vi "Power Output System Warning.vi"(6 "Driver Ref (null)":T10, 7 "Coerced PV Test Parameters":T1={"Stimulus"={"Frequency Type"=enum."Band Edges", "Frequency Ranges"=[], "TX 1 Frequency (MHz)"={"Min"=0.0, "Max"=0.0}, "TX 2 Frequency (MHz)"={"Min"=0.0, "Max"=0.0}, "RX Frequency (MHz)"={"Min"=0.0, "Max"=0.0}, "Pad Model Number"="", "Pad Serial Number"="", "Pad Values"=[]}, "Measurement"={"DUT Port"=enum."Port 1", "Direction"=0, "Frequency Step Size"=0}, "Display"={"Frequency"={"Min"=-1.0, "Max"=-1.0}, "Power"={"Min"=-1, "Max"=-1}}, "Limit"={"Min Power (dBm)"=44.0}, "Calibration"={"Calibrated?"=FALSE}} {"Measurement"."Frequency Step Size" items=["0.2", "0.4", "1.0", "2.0", "4.0"]; "Measurement"."Direction" items=["Reverse", "Forward", "Auxiliary"]}, 10 "PV Test Parameters":T1={"Stimulus"={"Frequency Type"=enum."Band Edges", "Frequency Ranges"=[], "TX 1 Frequency (MHz)"={"Min"=0.0, "Max"=0.0}, "TX 2 Frequency (MHz)"={"Min"=0.0, "Max"=0.0}, "RX Frequency (MHz)"={"Min"=0.0, "Max"=0.0}, "Pad Model Number"="", "Pad Serial Number"="", "Pad Values"=[]}, "Measurement"={"DUT Port"=enum."Port 1", "Direction"=0, "Frequency Step Size"=0}, "Display"={"Frequency"={"Min"=-1.0, "Max"=-1.0}, "Power"={"Min"=-1, "Max"=-1}}, "Limit"={"Min Power (dBm)"=44.0}, "Calibration"={"Calibrated?"=FALSE}} {"Measurement"."Frequency Step Size" items=["0.2", "0.4", "1.0", "2.0", "4.0"]; "Measurement"."Direction" items=["Reverse", "Forward", "Auxiliary"]}, 11 "TestSetDef":T11={"General"={"ID"=0, "Model"="", "Dual Port?"=FALSE, "Options"="", "Options"={"E"=FALSE, "K"=FALSE, "H"=FALSE, "W"=FALSE, "F"=FALSE}, "Cal File"=path ""}, "Receiver"={"Fstart, MHz"=0.0, "Fstop MHz"=0.0, "Fstep MHz"=0.0, "IF, MHz"=0.0}, "RX Band"={"Fstart, MHz"=0.0, "Fstop MHz"=0.0}, "TX 1"={"Fstart, MHz"=0.0, "Fstop MHz"=0.0, "Pmax, dBm"=0.0, "Pstep, dB"=0.0}, "TX 2"={"Fstart, MHz"=0.0, "Fstop MHz"=0.0, "Pmax, dBm"=0.0, "Pstep, dB"=0.0}, "Low-side?"=TRUE}) -> (2 "Message (\"\")":string="\n\n", 3 "Abort?":bool)   [LabVIEW 2011]
uses:
  SI.LIB/PIM.LIB/HW IO/Test Set Definition.ctl
  TypeDefs/Power Output Test Parameters.ctl
  TypeDefs/Power Output Stimulus Parameters.ctl
  TypeDefs/Power Output Measurement Parameters.ctl
  SI.LIB/PIM.LIB/HW IO/DUTport.ctl
  SI.LIB/PIM.LIB/HW IO/MeasMode.ctl
  SI.LIB/PIM.LIB/HW IO/PIM Sweep Step Size.ctl
  TypeDefs/Power Output Display Parameters.ctl
  TypeDefs/Power Output Limit Parameters.ctl
  TypeDefs/Power Output Calibration State.ctl
  drivers/PIM/PIM Driver Ref.ctl
  drivers/PIM/PIM Command.ctl
panel:
  in  "B 2":bool
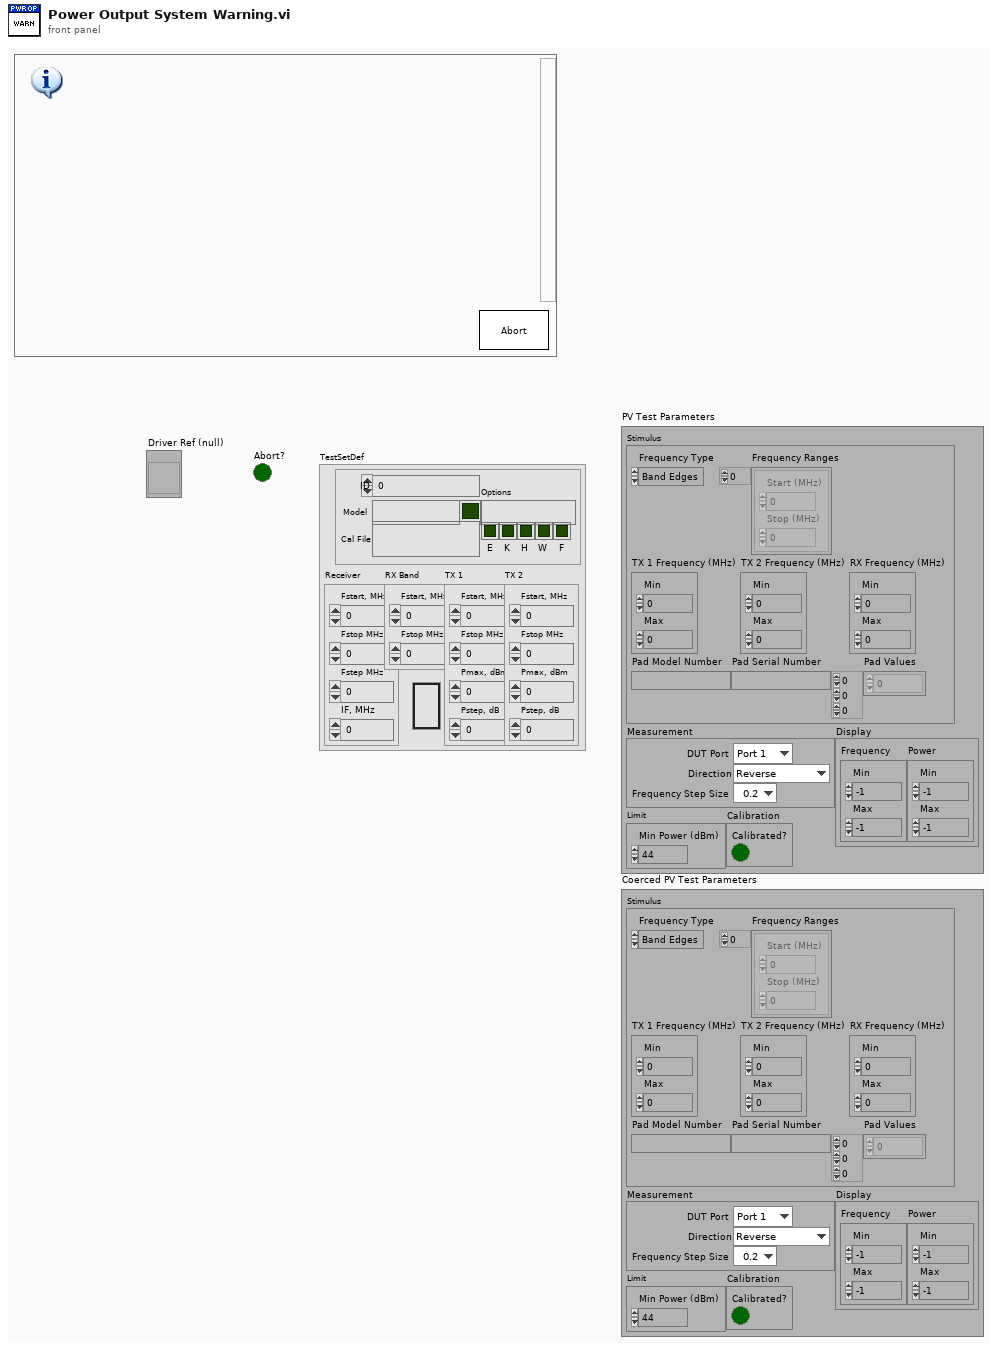
[diagram p1: front panel]
types:
  T1 = typedef "Power Output Test Parameters.ctl" = cluster{"Stimulus":T2, "Measurement":T3, "Display":T7, "Limit":T8, "Calibration":T9}
  T2 = typedef "Power Output Stimulus Parameters.ctl" = cluster{"Frequency Type":enum16{"Band Edges", "Custom"}, "Frequency Ranges":cluster{"Start (MHz)":dbl, "Stop (MHz)":dbl}[], "TX 1 Frequency (MHz)":cluster{"Min":dbl, "Max":dbl}, "TX 2 Frequency (MHz)":cluster{"Min":dbl, "Max":dbl}, "RX Frequency (MHz)":cluster{"Min":dbl, "Max":dbl}, "Pad Model Number":string, "Pad Serial Number":string, "Pad Values":dbl[][][]}
  T3 = typedef "Power Output Measurement Parameters.ctl" = cluster{"DUT Port":T4, "Direction":T5, "Frequency Step Size":T6}
  T4 = typedef "DUTport.ctl" = enum16{"Port 1", "Port 2"}
  T5 = typedef "MeasMode.ctl" = u16
  T6 = typedef "PIM Sweep Step Size.ctl" = u16
  T7 = typedef "Power Output Display Parameters.ctl" = cluster{"Frequency":cluster{"Min":dbl, "Max":dbl}, "Power":cluster{"Min":i32, "Max":i32}}
  T8 = typedef "Power Output Limit Parameters.ctl" = cluster{"Min Power (dBm)":dbl}
  T9 = typedef "Power Output Calibration State.ctl" = cluster{"Calibrated?":bool}
  T10 = typedef "PIM Driver Ref.ctl" = refnum<vi>
  T11 = typedef "Test Set Definition.ctl" = cluster{"General":cluster{"ID":u32, "Model":string, "Dual Port?":bool, "Options":string, "Options":cluster{"E":bool, "K":bool, "H":bool, "W":bool, "F":bool}, "Cal File":path}, "Receiver":cluster{"Fstart, MHz":dbl, "Fstop MHz":dbl, "Fstep MHz":dbl, "IF, MHz":dbl}, "RX Band":cluster{"Fstart, MHz":dbl, "Fstop MHz":dbl}, "TX 1":cluster{"Fstart, MHz":dbl, "Fstop MHz":dbl, "Pmax, dBm":dbl, "Pstep, dB":dbl}, "TX 2":cluster{"Fstart, MHz":dbl, "Fstop MHz":dbl, "Pmax, dBm":dbl, "Pstep, dB":dbl}, "Low-side?":bool}
  T12 = typedef "PIM Command.ctl" = enum16{"LOAD", "KEEP ALIVE", "VALIDATE", "INITIALIZE", "PRESET", "GET CALIBRATION", "SET STIMULUS", "TOGGLE TX POWER", "SET TX ON", "SET TX OFF", "MEASURE", "UNLOAD"}
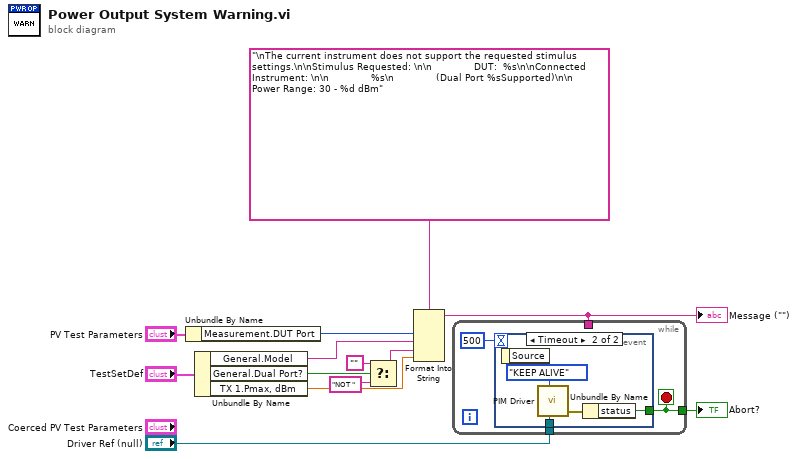
[diagram p0: block diagram]
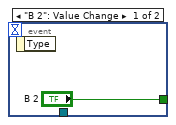
[diagram p2: hidden frame]
diagram:
  n1 = Unbundle By Name("PV Test Parameters") -> ("Measurement.DUT Port"=w3:T4)
  n2 = Unbundle By Name("TestSetDef") -> ("General.Model"=w11:string, "General.Dual Port?"=w6:bool, "TX 1.Pmax, dBm"=w2:dbl)
  n3 = Select(t="", s=w6, f="NOT " ("string")) -> (s? t:f=w1:string)
  n4 = Format Into String(format string="\nThe current instrument does not support the requested stimulus settings.\n\nStimulus Requested: \n\n              DUT:  %s\n\nConnected Instrument: \n\n              %s\n              (Dual Port %sSupported)\n\n              Power Range: 30 - %d dBm", w3, w11, w1, w2) -> (resulting string=w5:string)  [unwired: 2 in, 1 out]
  "Message (\"\")" <- w5
  n5 = while {
    tunnel: [w16] -> w13
    tunnel: w5 -> [_]
    tunnel: "Driver Ref (null)" -> [w14]
    stop <- w16 stop-if-true
    n6 = event shown="[1] Timeout" {
      selector: _ -> [_ _]
      dyn-events: _ -> [_ _]
      timeout: 500 -> [_ _]
      tunnel: ["B 2" w19] -> w16
      tunnel: w14 -> [_ w18]
      event "B 2": Value Change {
        n7 = event-data() -> ()  [unwired: 2 out]
      }
      event Timeout {
        n8 = event-data() -> ()  [unwired: 2 out]
        n9 = call "PIM Driver.vi"("Driver Ref (null)"=w18, "PIM Command"=PIM_Command."KEEP ALIVE") -> ("error out"=w20:errorcluster)  [unwired: 3 in, 6 out]
        n10 = Unbundle By Name(w20) -> ("status"=w19:bool)
      }
    }
  }
  "Abort?" <- w13
